vi "createServerStatusNotifier.vi"(8 "error in (no error)":errorcluster, 10 "notifierName (unnamed)":string, 11 "tcpServerBase in":refnum<class "TcpServerBase.lvclass">) -> (0 "error out":errorcluster, 3 "tcpServerBase out":refnum<class "TcpServerBase.lvclass">)   [LabVIEW 2018]
doc: "Create serverStatusNotifier reference to send a notification from TCP Server to User everytime TCP Client connects or disconnects. \n\nIf the notifierName control is empty the default empty string will be added to the name."
uses:
  TcpServerBase.lvclass
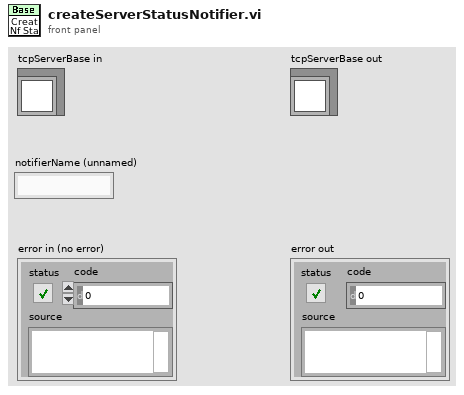
[diagram p1: front panel]
types:
  T1 = cluster{"connectionStatus":bool, "errorSource":string}
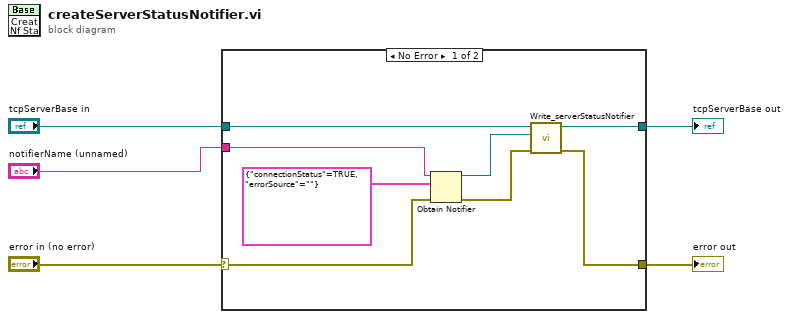
[diagram p0: block diagram]
diagram:
  n1 = case shown="No Error" "error in (no error)" {
    selector: "error in (no error)" -> [w12 w15]
    tunnel: "tcpServerBase in" -> [w11 w14]
    tunnel: [w8 w14] -> w4
    tunnel: [w7 w15] -> w2
    tunnel: "notifierName (unnamed)" -> [w6 _]
    frame No Error {
      n2 = Obtain Notifier(name (unnamed)=w6, notification data type=T1 {"connectionStatus"=TRUE, "errorSource"=""}, error in (no error)=w12) -> (notifier out=w9:refnum<notifier>, error out=w10:errorcluster)  [unwired: 1 in, 1 out]
      n3 = call "Write_serverStatusNotifier.vi"("error in (no error)"=w10, "serverStatusNotifier"=w9, "TcpServerBase in"=w11) -> ("error out"=w7:errorcluster, "TcpServerBase out"=w8:refnum<class "TcpServerBase.lvclass">)  [unwired: 7 in]
    }
    frame Error {
    }
  }
  "error out" <- w2
  "tcpServerBase out" <- w4
